vi "LCA Get Axis System Axis Number.vi"(8 "error in (no error)":errorcluster caption="Fehler (Eingang, kein Fehler)", 11 "Axis System Handle":i64) -> (0 "error out":errorcluster caption="Fehler (Ausgang)", 3 "Axis Count":i32)   [LabVIEW 2021, in "labbCAN_MotionControl_API.lvlib"]
doc: "LCA_Func dev_hdl __stdcall LCA_GetAxisSystemAxisNumber(dev_hdl hAxisSystem);"
uses:
  labbCAN_MotionControl_API.lvlib
  labbCAN_MotionControl_API.dll
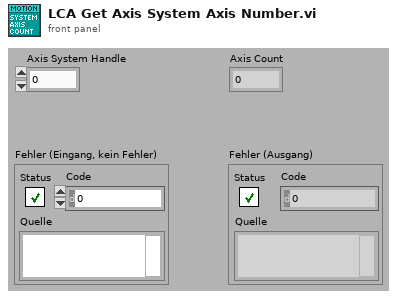
[diagram p1: front panel]
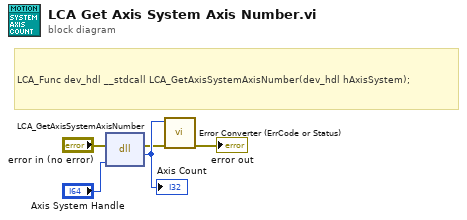
[diagram p0: block diagram]
diagram:
  # "LCA_Func dev_hdl __stdcall LCA_GetAxisSystemAxisNumber(dev_hdl hAxisSystem);"
  n1 = dll-call lib="C:/Users/olaja/AppData/Local/CETONI_SDK/labbCAN_MotionControl_API.*" fn="LCA_GetAxisSystemAxisNumber"(error in="error in (no error)", "hAxisSystem"="Axis System Handle") -> (error out=w2:errorcluster, "Rückgabetyp"=w5:i32)  [unwired: 3 in, 1 out]
  "Axis Count" <- w5
  n2 = call "Error Converter (ErrCode or Status).vi"("error in (no error)"=w2, "error code"=w5) -> ("error out"=→"error out":errorcluster)  [unwired: 9 in]
